vi "Reset TD4.vi"(8 "error in (no error)":errorcluster, 11 "TD4 in":refnum<class "TD4.lvclass">) -> (0 "error out":errorcluster, 3 "TD4 out":refnum<class "TD4.lvclass">)   [LabVIEW 2025, in "TD4.lvclass"]
uses:
  TD4.lvclass
  TD4.lvclass/TD4.ctl
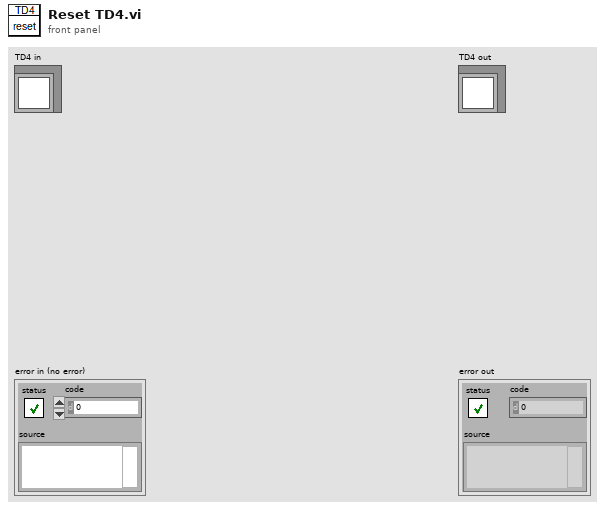
[diagram p1: front panel]
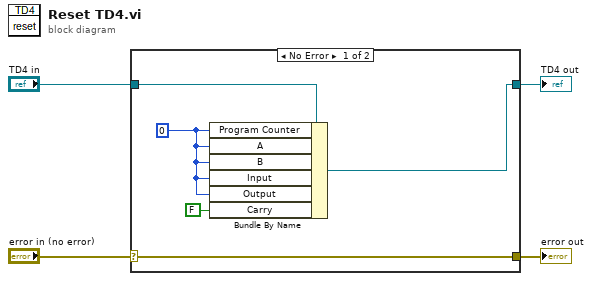
[diagram p0: block diagram]
diagram:
  n1 = case shown="No Error" "error in (no error)" {
    selector: "error in (no error)" -> [w9 w10]
    tunnel: [w9 w10] -> w3
    tunnel: [w7 w11] -> w1
    tunnel: "TD4 in" -> [w8 w11]
    frame No Error {
      w6 = u8 0 ("Program Counter")
      n2 = Bundle By Name(cluster=w8, "Program Counter"=w6, "A"=w6, "B"=w6, "Input"=w6, "Output"=w6, "Carry"=FALSE) -> (w7:refnum<class "TD4.lvclass">)
    }
    frame Error {
    }
  }
  "error out" <- w3
  "TD4 out" <- w1
